vi "Read DAQmx Configuration.vi"(8 "error in (no error)":errorcluster, 11 "DAQmx Recorder in":refnum<class "DAQmx Recorder.lvclass">) -> (0 "error out":errorcluster, 2 "Configuration":T1={"Pre-trigger duration"=0.01, "Post-trigger duration"=0.1, "Rate"=1000000.0, "Range"=10.0, "Physical Channels"="", "input configuration"=-1} {"input configuration" items=["Default"=-1, "RSE"=10083, "NRSE"=10078, "Differential"=10106, "Pseudodifferential"=12529]; "Rate" format="%#_6pHz"; "Post-trigger duration" format="%#_6ps"; "Pre-trigger duration" format="%#_6ps"; "Range" format="%#_6pV"}, 3 "DAQmx Recorder out":refnum<class "DAQmx Recorder.lvclass">)   [LabVIEW 2015, in "DAQmx Recorder.lvclass"]
uses:
  DAQmx Recorder.lvclass
  NHMFL_Core/Libraries/NI-DAQ/DAQmx Digitizer/DAQmx Digitizer Configuration.ctl
  Measure_core/Measure Object/Measure Object.lvclass/Measure Object.ctl
  Measure_core/Measure Object/Read Configuration.vi
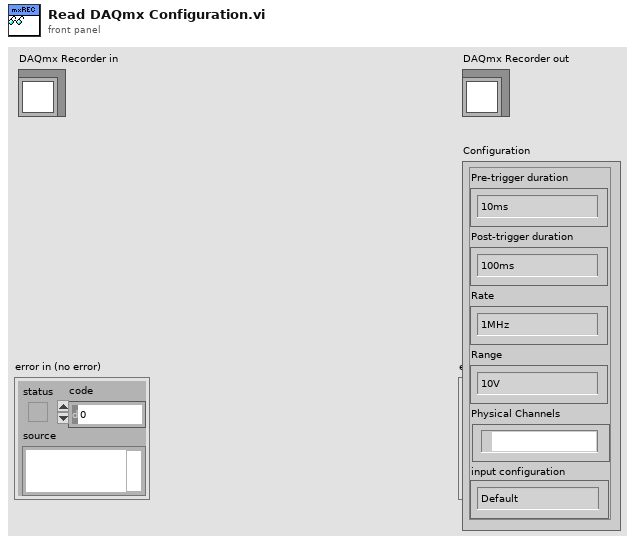
[diagram p1: front panel]
types:
  T1 = typedef "DAQmx Digitizer Configuration.ctl" = cluster{"Pre-trigger duration":dbl, "Post-trigger duration":dbl, "Rate":dbl, "Range":dbl, "Physical Channels":tag, "input configuration":i32}
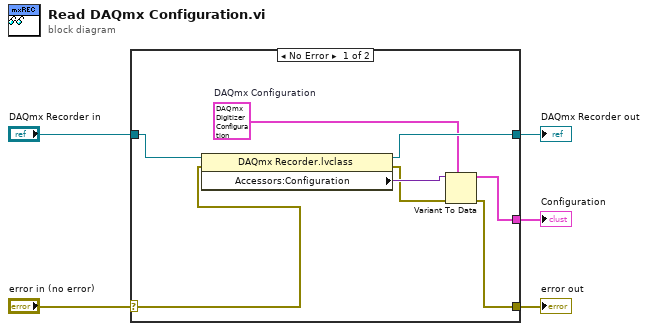
[diagram p0: block diagram]
diagram:
  n1 = case shown="No Error" "error in (no error)" {
    selector: "error in (no error)" -> [w7 w14]
    tunnel: [w8 w14] -> w4
    tunnel: [w12 w15] -> w2
    tunnel: "DAQmx Recorder in" -> [w13 w15]
    tunnel: [w6 _] -> w1
    frame No Error {
      w11 = T1 {"Pre-trigger duration"=0.01, "Post-trigger duration"=0.1, "Rate"=1000000.0, "Range"=10.0, "Physical Channels"="", "input configuration"=-1}  # DAQmx Configuration
      n2 = property class="DAQmx Recorder.lvclass"(reference=w13, error in=w7) -> (reference out=w12:refnum<class "DAQmx Recorder.lvclass">, error out=w9:errorcluster, "Accessors:Configuration"=w10:variant)
      n3 = Variant To Data(error in=w9, type=w11, Variant=w10) -> (data=w6:T1, error out=w8:errorcluster)
    }
    frame Error {
    }
  }
  "error out" <- w4
  "DAQmx Recorder out" <- w2
  "Configuration" <- w1
